vi "divider.vi"(11 "动作":string) -> (2 "方向":string, 3 "动作 out":string)   [LabVIEW 2014, in "Dialogue.lvlib" / "Dialogue.lvclass"]
uses:
  Dialogue.lvclass
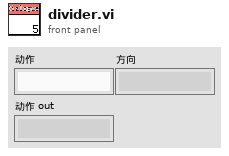
[diagram p1: front panel]
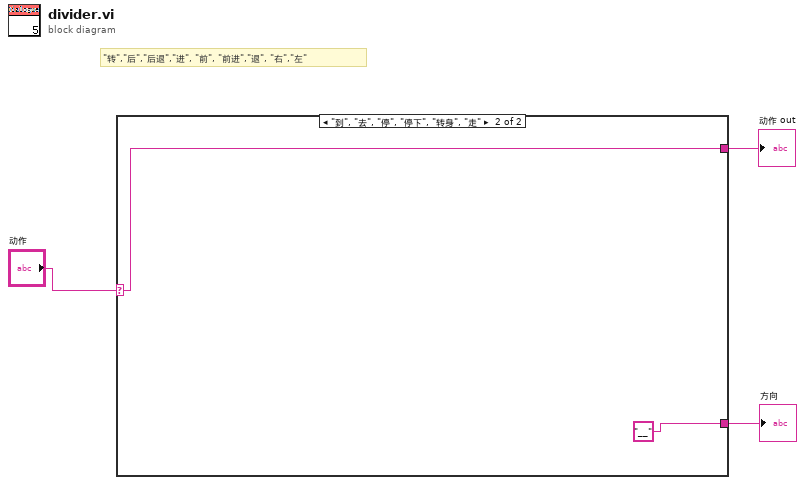
[diagram p0: block diagram]
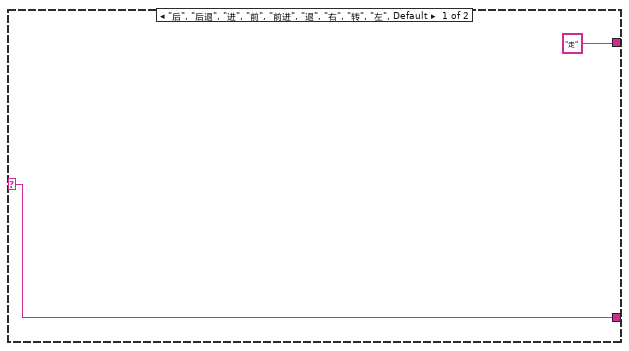
[diagram p2: hidden frame]
diagram:
  # "\"转\",\"后\",\"后退\",\"进\", \"前\", \"前进\",\"退\", \"右\",\"左\""
  n1 = case shown="\"到\", \"去\", \"停\", \"停下\", \"转身\", \"走\"" "动作" {
    selector: "动作" -> [w5 w6]
    tunnel: [w5 "__" ("起点")] -> w2
    tunnel: ["走" ("起点") w6] -> w1
    frame "后", "后退", "进", "前", "前进", "退", "右", "转", "左", Default {
    }
    frame "到", "去", "停", "停下", "转身", "走" {
    }
  }
  "动作 out" <- w1
  "方向" <- w2
